vi "Interp Test.vi"() -> ()   [LabVIEW 2012]
doc: "This example shows the operation of the 1D interpolation VI using three selectable test sets."
uses:
  Magna Power Constants.vi
  <vilib>/gmath/NI_Gmath.lvlib
panel:
  in  "stop":bool
  in  "Tab Control":enum32{"Graph", "Data"}(tab)
  out "1D Interpolation Graph":cluster{"yi":dbl[], "ramp data":dbl[]}[](graph)
  out "Interpolated Data":dbl[][](array[numeric])
  out "Original Data":dbl[][](array[numeric])
  in  "Method":i32(ring)=2 items=["nearest", "linear", "spline", "cubic Hermite", "Lagrange"]
  in  "Data Sets":enum16{"Test Set 1", "Test Set 2", "Test Set 3"}(ring)
  # "The following example shows the operation of the 1D interpolation VI using three selectable test sets.\n\nInstructions:\n1) Run the VI\n2) Modify the Data Sets and interpolation Method, and view the results on both the Graph and Data tabs\n3) Stop the VI and look at the Block Diagram for more information"
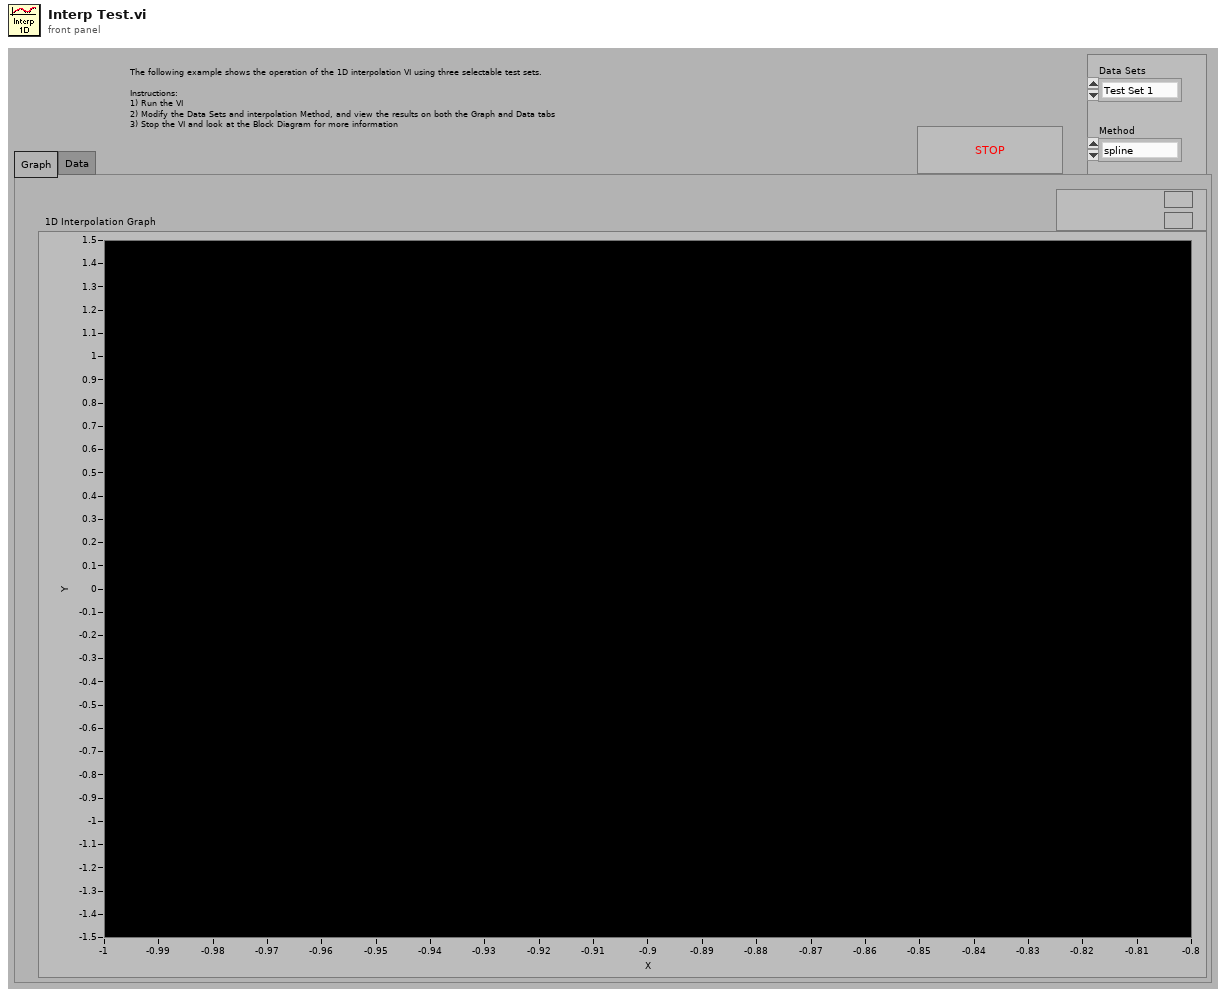
[diagram p1: front panel]
types:
  T1 = cluster{"starting value":dbl, "increment":dbl, "final value":dbl}
  T2 = cluster{"Fluke Voltages":dbl[], "Field Values":dbl[]}
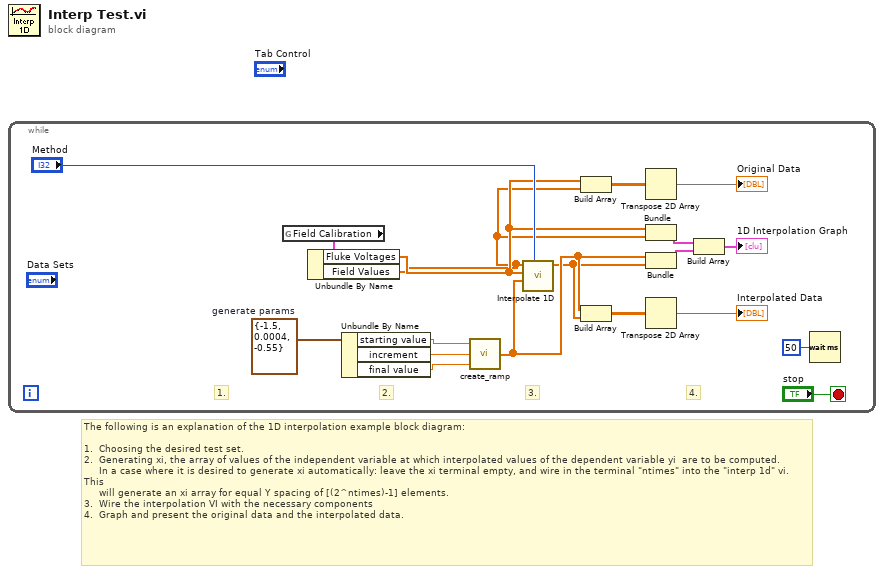
[diagram p0: block diagram]
diagram:
  # "The following is an explanation of the 1D interpolation example block diagram:\n\n1.  Choosing the desired test set.\n2.  Generating xi, the array of values of the independent variable at which interpolated values of the dependent variable yi  are to be computed. \n     In a case where it is desired to generate xi automatically: leave the xi terminal empty, and wire in the terminal \"ntimes\" into the \"interp 1d\" vi.  This\n     will generate an xi array for equal Y spacing of [(2^ntimes)-1] elements.\n3.  Wire the interpolation VI with the necessary components\n4.  Graph and present the original data and the interpolated data."
  n1 = while {
    stop <- "stop" stop-if-true
    w3 = T1 {"starting value"=-1.5, "increment"=0.0004, "final value"=-0.55}  # generate params
    # "4."
    # "3."
    # "2."
    # "1."
    n2 = global read "Magna Power Constants.vi" "Field Calibration"() -> (w4:T2)
    n3 = Unbundle By Name(w4) -> ("Fluke Voltages"=w2:dbl[], "Field Values"=w1:dbl[])
    n4 = Unbundle By Name(w3) -> ("starting value"=w14:dbl, "increment"=w13:dbl, "final value"=w12:dbl)
    n5 = call "create_ramp.vi"("final value"=w12, "increment"=w13, "starting value"=w14) -> ("ramp data"=w8:dbl[])
    n6 = call <vilib>:"Interpolate 1D.vi"("method"="Method", "xi"=w8, "X"=w2, "Y"=w1) -> ("yi"=w7:dbl[])  [unwired: 5 in, 2 out]
    n7 = Build Array(w2, w1) -> (w11:dbl[][])
    n8 = Build Array(w8, w7) -> (w9:dbl[][])
    n9 = Transpose 2D Array(2D array=w11) -> (transposed array=→"Original Data":dbl[][])
    n10 = Bundle("Fluke Voltages"=w2, "Field Values"=w1) -> (w16:T2)  [unwired: 1 in]
    n11 = Bundle("ramp data"=w8, "yi"=w7) -> (w17:cluster{"ramp data":dbl[], "yi":dbl[]})  [unwired: 1 in]
    n12 = Transpose 2D Array(2D array=w9) -> (transposed array=→"Interpolated Data":dbl[][])
    n13 = Build Array(w16, w17) -> (→"1D Interpolation Graph":cluster{"ramp data":dbl[], "yi":dbl[]}[])
    n14 = Wait (ms)(milliseconds to wait=u32 50) -> ()  [unwired: 1 out]
  }
